vi "UI Populate Label List.vi"(8 "error in (no error)":errorcluster, 11 "Controller in":refnum<class "Controller.lvclass">) -> (0 "error out":errorcluster, 3 "Controller out":refnum<class "Controller.lvclass">)   [LabVIEW 2013, in "SET Project Editor.lvlib" / "Controller.lvclass"]
uses:
  Controller.lvclass
  Controller.lvclass/Controller.ctl
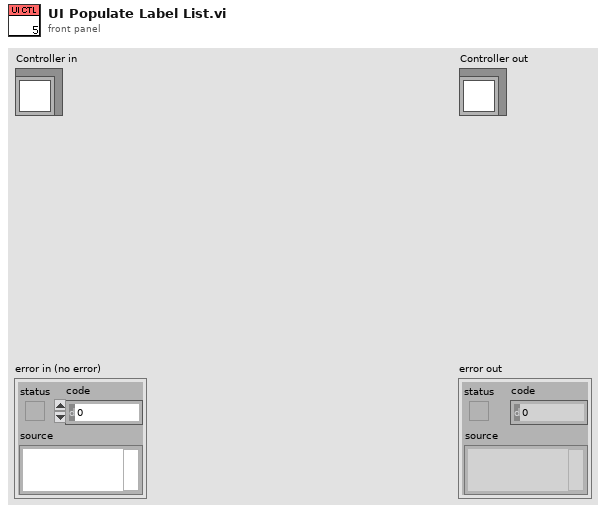
[diagram p1: front panel]
types:
  T1 = cluster{"Left Cell String":string, "Child Text":string[], "Child Tag":string, "Item Indent":i32, "Child Only?":bool, "Glyph Index":i32}[]
  T2 = cluster{"Left Cell String":string, "Child Text":string[], "Child Tag":string, "Item Indent":i32, "Child Only?":bool, "Glyph Index":i32}
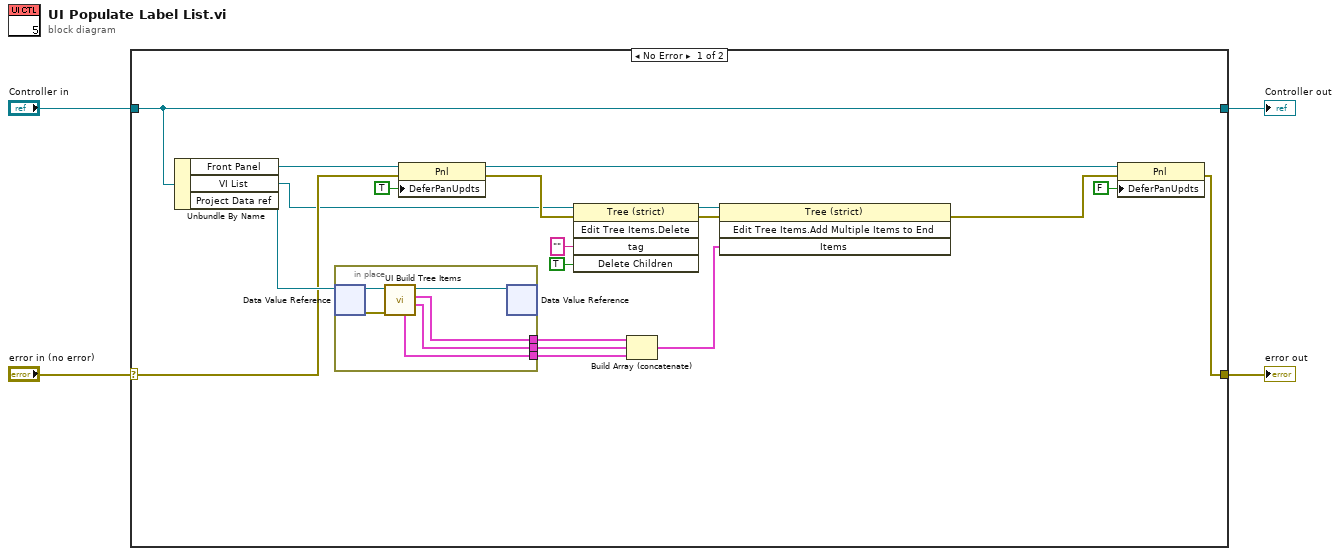
[diagram p0: block diagram]
diagram:
  n1 = case shown="No Error" "error in (no error)" {
    selector: "error in (no error)" -> [w19 w31]
    tunnel: [w11 w31] -> w3
    tunnel: [w23 w30] -> w1
    tunnel: "Controller in" -> [w23 w30]
    frame No Error {
      n2 = Unbundle By Name(w23) -> ("Front Panel"=w18:refnum<vi>, "VI List"=w12:refnum<vi>, "Project Data ref"=w22:refnum<data-value>)
      n3 = in-place {
        in-place-border: [w26] -> w8
        in-place-border: [w25] -> w6
        in-place-border: [w24] -> w5
        n4 = in-place-dvr #1(w22) -> (w29:refnum<class "Project Data.lvclass">, w27:errorcluster)
        n5 = call "UI Build Tree Items.vi"("error in (no error)"=w27, "LangData in"=w29) -> ("RTM List"=w25:T1, "VI List"=w26:T1, "LangData out"=w28:refnum<class "Project Data.lvclass">, "SR List"=w24:T2)  [unwired: 5 in, 1 out]
        n6 = in-place-dvr #1(w28) -> ()  [unwired: 2 out]
      }
      n7 = property class="Pnl"(reference=w18, error in=w19, "DeferPanUpdts"=TRUE ("Defer Panel Updates")) -> (reference out=w10:refnum<vi>, error out=w13:errorcluster)
      n8 = invoke class="Tree (strict)" method="Edit Tree Items.Delete"(reference=w12, error in=w13, "tag"="" ("Tag"), "Delete Children"=TRUE ("Delete Children?")) -> (reference out=w16:refnum<vi>, error out=w17:errorcluster)  [unwired: 1 in, 3 out]
      n9 = Build Array (concatenate)(w8, w6, w5) -> (w7:T1)
      n10 = invoke class="Tree (strict)" method="Edit Tree Items.Add Multiple Items to End"(reference=w16, error in=w17, "Items"=w7) -> (error out=w9:errorcluster)  [unwired: 1 in, 3 out]
      n11 = property class="Pnl"(reference=w10, error in=w9, "DeferPanUpdts"=FALSE ("Defer Panel Updates")) -> (error out=w11:errorcluster)  [unwired: 1 out]
    }
    frame Error {
    }
  }
  "error out" <- w3
  "Controller out" <- w1
